vi "ort_fit_accWeights.vi"() -> (0 "Init Data Out":fxp<+,18,0>[](array[numeric]))   [LabVIEW 2016]
panel:
  # "For Initialization VI requirements and help, please read directions located on Block Diagram."
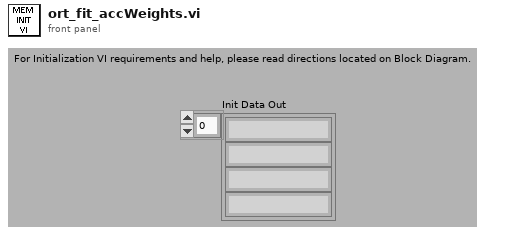
[diagram p1: front panel]
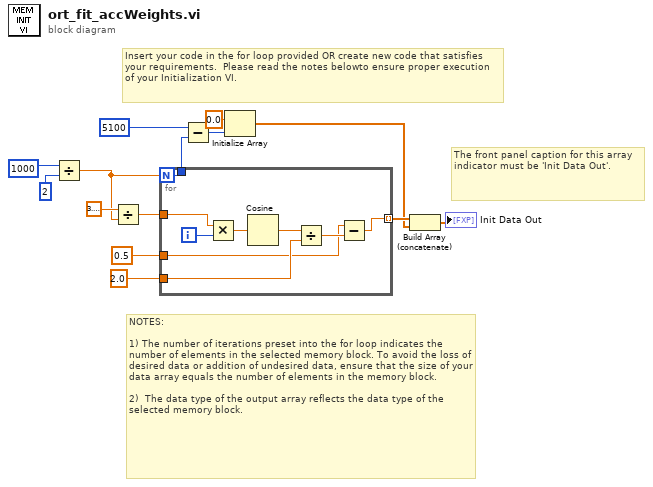
[diagram p0: block diagram]
diagram:
  # "The front panel caption for this array indicator must be 'Init Data Out'."
  # "NOTES:\n\n1) The number of iterations preset into the for loop indicates the number of elements in the selected memory block. To avoid the loss of desired data or addition of undesired data, ensure that the size of your data array equals the number of elements in the memory block.\n\n2)  The data type of the output array reflects the data type of the selected memory block."
  # "Insert your code in the for loop provided OR create new code that satisfies your requirements.  Please read the notes belowto ensure proper execution of your Initialization VI."
  n1 = Divide(x=1000 ("Number of Elements"), y=2) -> (x/y=w7:dbl)
  n2 = Divide(x=3.141592653589793, y=w7) -> (x/y=w13:dbl)
  n3 = for {
    N: w7 -> [w16]
    tunnel: [w15] -> w4 mode=indexing
    tunnel: w13 -> [w20]
    tunnel: 2.0 ("y") -> [w18]
    tunnel: 0.5 ("x") -> [w17]
    tunnel: [w16] -> w5
    i -> [w19]
    n4 = Multiply(x=w20, y=w19) -> (x*y=w23:dbl)
    n5 = Cosine(x=w23) -> (cos(x)=w22:dbl)
    n6 = Divide(x=w22, y=w18) -> (x/y=w21:dbl)
    n7 = Subtract(x=w17, y=w21) -> (x-y=w15:dbl)
  }
  n8 = Subtract(x=5100 ("Number of Elements"), y=w5) -> (x-y=w6:i32)
  n9 = Initialize Array(0.0 ("element"), w6) -> (w1:dbl[])
  n10 = Build Array (concatenate)(w4, w1) -> (→"Init Data Out":dbl[])
